vi "draw_circle_on_graph.vi"(10 "半径R":dbl, 11 "プロット数N":dbl) -> (3 "XYグラフ":cluster{dbl[], dbl[]}(graph))   [LabVIEW 2020]
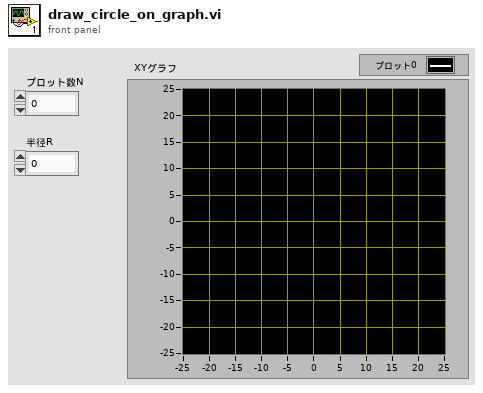
[diagram p1: front panel]
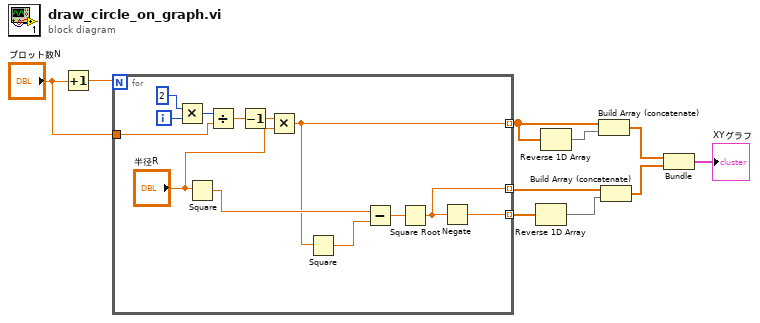
[diagram p0: block diagram]
diagram:
  n1 = Increment(x="プロット数N") -> (x+1=w10:dbl)
  n2 = for {
    N: w10 -> [_]
    tunnel: [w14] -> w8 mode=indexing
    tunnel: [w13] -> w2 mode=indexing
    tunnel: "プロット数N" -> [w12]
    tunnel: [w11] -> w4 mode=indexing
    i -> [w21]
    n3 = Multiply(x=2, y=w21) -> (x*y=w19:i32)
    n4 = Square(x="半径R") -> (x^2=w23:dbl)
    n5 = Divide(x=w19, y=w12) -> (x/y=w18:dbl)
    n6 = Decrement(x=w18) -> (x-1=w17:dbl)
    n7 = Multiply(x=w17, y="半径R") -> (x*y=w11:dbl)
    n8 = Square(x=w11) -> (x^2=w15:dbl)
    n9 = Subtract(x=w23, y=w15) -> (x-y=w22:dbl)
    n10 = Square Root(x=w22) -> (sqrt(x)=w14:dbl)
    n11 = Negate(x=w14) -> (-x=w13:dbl)
  }
  n12 = Reverse 1D Array(array=w2) -> (reversed array=w1:dbl[])
  n13 = Reverse 1D Array(array=w4) -> (reversed array=w3:dbl[])
  n14 = Build Array (concatenate)(w4, w3) -> (w7:dbl[])
  n15 = Build Array (concatenate)(w8, w1) -> (w6:dbl[])
  n16 = Bundle(w7, w6) -> (→"XYグラフ":cluster{dbl[], dbl[]})  [unwired: 1 in]
